vi "Shooter Speed Up.vi"(11 "Shooter P":dbl) -> (3 "Shooter Output":dbl)   [LabVIEW 2016]
uses:
  Robot Global Data.vi
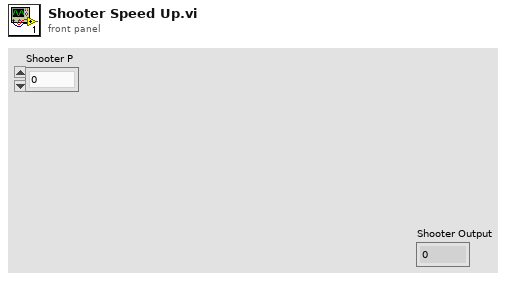
[diagram p1: front panel]
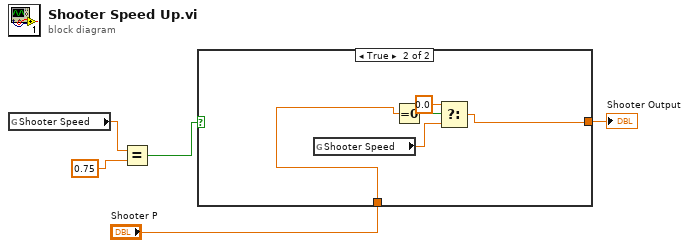
[diagram p0: block diagram]
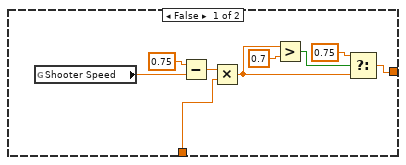
[diagram p2: hidden frame]
diagram:
  n1 = global read "Robot Global Data.vi" "Shooter Speed"() -> (w4:dbl)
  n2 = Equal?(x=w4, y=0.75 ("x")) -> (x = y?=w2:bool)
  n3 = case shown="True" w2 {
    tunnel: [w7 w16] -> w5
    tunnel: "Shooter P" -> [w6 w15]
    frame False {
      n4 = global read "Robot Global Data.vi" "Shooter Speed"() -> (w14:dbl)
      n5 = Subtract(x=0.75, y=w14) -> (x-y=w12:dbl)
      n6 = Multiply(x=w12, y=w6) -> (x*y=w8:dbl)
      n7 = Greater?(x=w8, y=0.7) -> (0:w11:bool)
      n8 = Select(t=0.75, s=w11, f=w8) -> (s? t:f=w7:dbl)
    }
    frame True {
      n9 = global read "Robot Global Data.vi" "Shooter Speed"() -> (w17:dbl)
      n10 = Equal To 0?(x=w15) -> (x = 0?=w19:bool)
      n11 = Select(t=0.0, s=w19, f=w17) -> (s? t:f=w16:dbl)
    }
  }
  "Shooter Output" <- w5
